vi "Some VI 3.vi"(8 "Error In":errorcluster) -> (0 "Error Out":errorcluster, 2 "signal out 2":waveform(dbl))   [LabVIEW 2014]
uses:
  <vilib>/measure/NI_MABase.lvlib
panel:
  out "signal out":waveform(dbl)
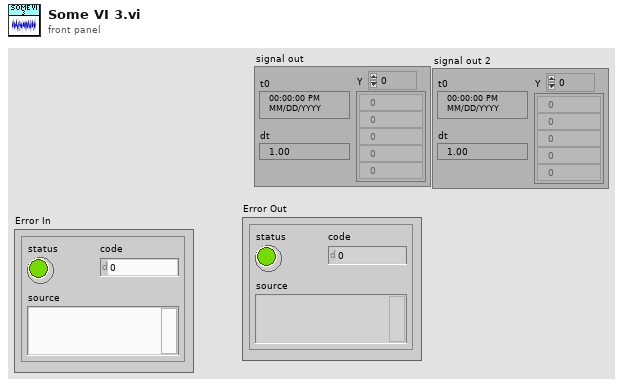
[diagram p1: front panel]
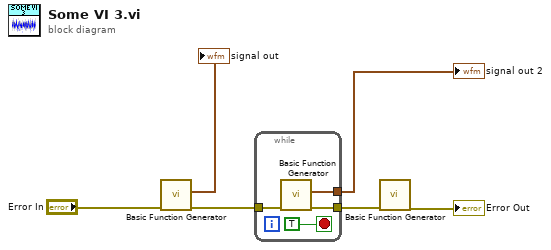
[diagram p0: block diagram]
diagram:
  n1 = call <vilib>:"Basic Function Generator.vi"("error in (no error)"="Error In") -> ("error out"=w5:errorcluster, "signal out"=→"signal out":waveform(dbl))  [unwired: 8 in, 1 out]
  n2 = while {
    tunnel: [w8] -> w3
    tunnel: w5 -> [w10]
    tunnel: [w9] -> w2
    stop <- TRUE stop-if-true
    n3 = call <vilib>:"Basic Function Generator.vi"("error in (no error)"=w10) -> ("error out"=w9:errorcluster, "signal out"=w8:waveform(dbl))  [unwired: 8 in, 1 out]
  }
  "signal out 2" <- w3
  n4 = call <vilib>:"Basic Function Generator.vi"("error in (no error)"=w2) -> ("error out"=→"Error Out":errorcluster)  [unwired: 8 in, 2 out]
